vi "Define RF Filter.vi"(8 "Error In":errorcluster, 9 "Filter Definition":T1={"Upper Cutoff [Hz]"=10000000.0, "Lower Cutoff [Hz]"=1000000.0, "Order"=1, "Type"=enum."Bandpass"} {"Upper Cutoff [Hz]" min=100000.0 max=100000000.0 step=100000.0 format="%#_6p"; "Lower Cutoff [Hz]" min=100000.0 max=100000000.0 step=100000.0 format="%#_6p"}, 10 "Sample Rate [1/s]":dbl=100000000.0 format="%#_6p") -> (0 "Error Out":errorcluster, 3 "IIR Filter Coefficients":T2)   [LabVIEW 2019]
uses:
  RF Filter Control.ctl
  <vilib>/Analysis/3filter.llb/Filter Passband Type.ctl
  <vilib>/Analysis/3filter.llb/Filter Structure Type.ctl
  <vilib>/Analysis/NI_AALBase.lvlib
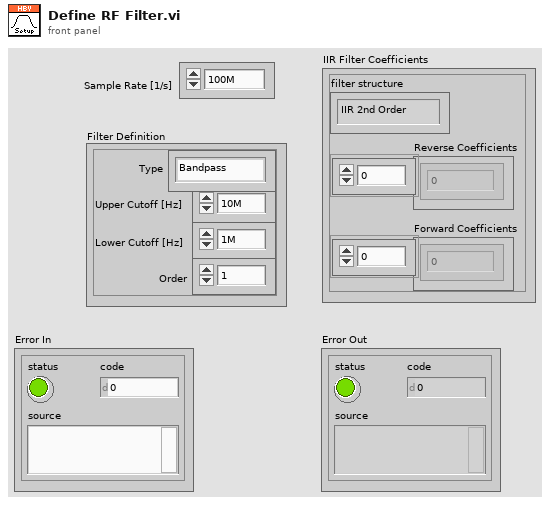
[diagram p1: front panel]
types:
  T1 = typedef "RF Filter Control.ctl" = cluster{"Upper Cutoff [Hz]":dbl, "Lower Cutoff [Hz]":dbl, "Order":i32, "Type":enum16{"Bandpass", "AC", "No Filter"}}
  T2 = cluster{"filter structure":enum32{"IIR 2nd Order", "IIR 4th Order"}, "Reverse Coefficients":dbl[], "Forward Coefficients":dbl[]}
  T3 = typedef "NI_AALBase.lvlib/Filter Structure Type.ctl" = u16
  T4 = typedef "NI_AALBase.lvlib/Filter Passband Type.ctl" = enum32{"Lowpass", "Highpass", "Bandpass", "Bandstop"}
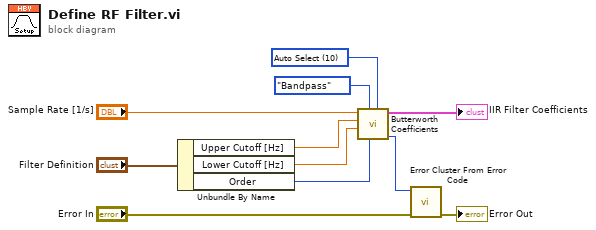
[diagram p0: block diagram]
diagram:
  w2 = T3 10 items=["IIR 2nd Order"=0, "IIR 4th Order"=1, "Auto Select"=10] ("filter structure option")
  n1 = Unbundle By Name("Filter Definition") -> ("Upper Cutoff [Hz]"=w6:dbl, "Lower Cutoff [Hz]"=w5:dbl, "Order"=w4:i32)
  n2 = call <vilib>:"Butterworth Coefficients.vi"("filter structure option"=w2, "order"=w4, "filter type"=Filter_Passband_Type."Bandpass", "low cutoff freq: fl"=w5, "high cutoff freq: fh"=w6, "sampling freq: fs"="Sample Rate [1/s]") -> ("error"=w11:i32, "IIR Filter Cluster"=→"IIR Filter Coefficients":T2)  [unwired: 4 in]
  n3 = call <vilib>:"Error Cluster From Error Code.vi"("error in (no error)"="Error In", "error code (0)"=w11) -> ("error out"=→"Error Out":errorcluster)  [unwired: 7 in]
